vi "GetTunnels.vi"(6 "error in":errorcluster, 9 "Structure in":refnum<class "Structure.lvclass">) -> (0 "error out":errorcluster, 3 "Structure out":refnum<class "Structure.lvclass">, 4 "Tunnels":i32[](array[numeric]))   [LabVIEW 2014, in "Structure.lvclass"]
uses:
  Structure.lvclass
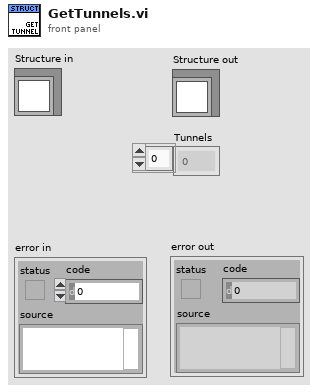
[diagram p1: front panel]
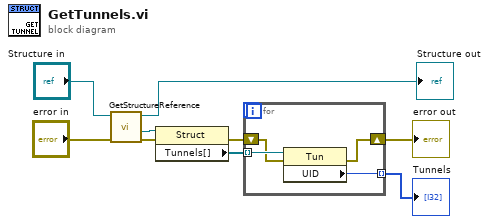
[diagram p0: block diagram]
diagram:
  n1 = call "GetStructureReference.vi"("error in"="error in", "Structure in"="Structure in") -> ("error out"=w7:errorcluster, "reference out"=w6:refnum<vi>, "Structure out"=→"Structure out":refnum<class "Structure.lvclass">)  [unwired: 7 in]
  n2 = property class="Struct"(reference=w6, error in=w7) -> (error out=w3:errorcluster, "Tunnels[]"=w4:refnum<vi>[])  [unwired: 1 out]
  n3 = for {
    tunnel: w4 -> [w13] mode=indexing
    tunnel: [w12] -> w1 mode=indexing
    shift-right: [w10] -> w2
    shift-left: w3 -> [w11]
    n4 = property class="Tun"(reference=w13, error in=w11) -> (error out=w10:errorcluster, "UID"=w12:i32)  [unwired: 1 out]
  }
  "error out" <- w2
  "Tunnels" <- w1
